vi "PID Open Loop Estimation.vi"(6 "CL Time Constant (T) 2":dbl, 7 "Controller Gain (K)":dbl, 9 "Dead Time (L)":dbl, 10 "CL Time Constant (Tcl)":dbl, 11 "CL Gain (Kcl)":dbl) -> (1 "Dead Time (L) Out":dbl, 2 "OL Time Constant (T)":dbl, 3 "OL Gain (Kp)":dbl)   [LabVIEW 2017, in "NI_PID_autopid.lvlib"]
uses:
  <vilib>/addons/control/pid/NI_PID_autopid.lvlib
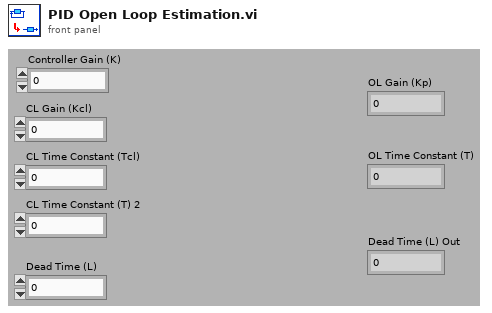
[diagram p1: front panel]
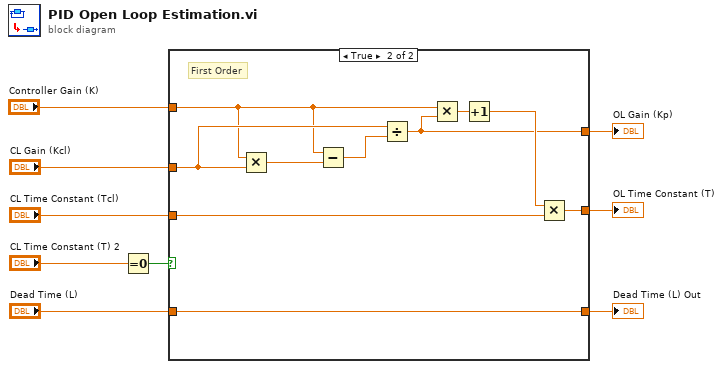
[diagram p0: block diagram]
diagram:
  n1 = Equal To 0?(x="CL Time Constant (T) 2") -> (x = 0?=w8:bool)
  n2 = case shown="True" w8 {
    tunnel: "CL Gain (Kcl)" -> [_ w19]
    tunnel: "CL Time Constant (Tcl)" -> [_ w15]
    tunnel: "Dead Time (L)" -> [_ w10]
    tunnel: "Controller Gain (K)" -> [_ w11]
    tunnel: [_ w13] -> w3
    tunnel: [_ w14] -> w2
    tunnel: [_ w10] -> w1
    frame False {
    }
    frame True {
      # "First Order"
      n3 = Multiply(x=w11, y=w19) -> (x*y=w17:dbl)
      n4 = Subtract(x=w11, y=w17) -> (x-y=w18:dbl)
      n5 = Divide(x=w19, y=w18) -> (x/y=w13:dbl)
      n6 = Multiply(x=w11, y=w13) -> (x*y=w12:dbl)
      n7 = Increment(x=w12) -> (x+1=w16:dbl)
      n8 = Multiply(x=w16, y=w15) -> (x*y=w14:dbl)
    }
  }
  "OL Gain (Kp)" <- w3
  "Dead Time (L) Out" <- w1
  "OL Time Constant (T)" <- w2
